vi "Convert String To Ring.vi"(8 "error in (no error)":errorcluster, 10 "Value":string, 11 "Ring Refnum":refnum<vi>) -> (0 "error out":errorcluster)   [LabVIEW 2013]
panel:
  in  "Numeric":u32
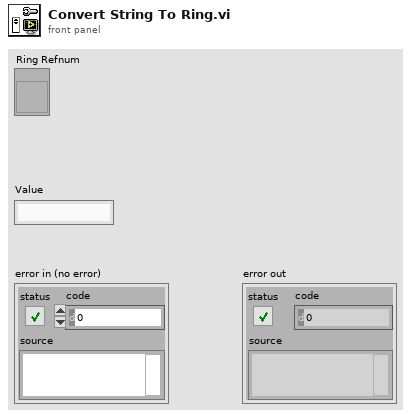
[diagram p1: front panel]
types:
  T1 = typedef "LVStringsAndValuesArrayTypeDef.ctl" = cluster{"String":string, "Value":ext}[]
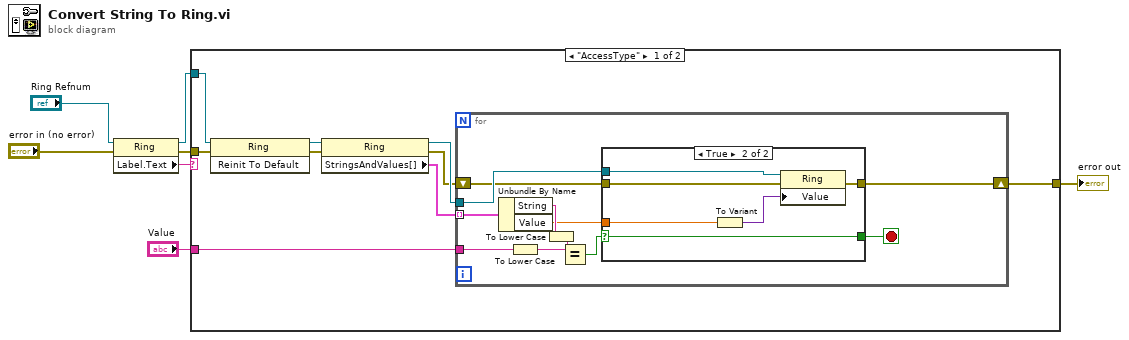
[diagram p0: block diagram]
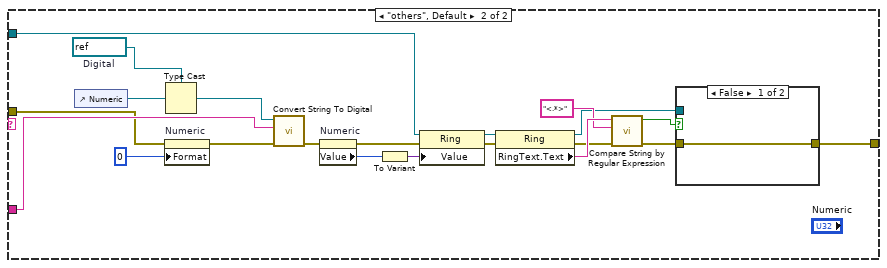
[diagram p3: hidden frame]
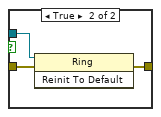
[diagram p4: hidden frame]
diagram:
  n1 = property class="Ring"(reference="Ring Refnum", error in="error in (no error)") -> (reference out=w4:refnum<vi>, error out=w2:errorcluster, "Label.Text"=w1:string)
  n2 = case shown="\"AccessType\"" w1 {
    tunnel: "Value" -> [w15 w56]
    tunnel: [w8 w43] -> w7
    tunnel: w2 -> [w13 w38]
    tunnel: w4 -> [w14 w36]
    frame "AccessType" {
      n3 = invoke class="Ring" method="Reinit To Default"(reference=w14, error in=w13) -> (reference out=w11:refnum<vi>, error out=w12:errorcluster)  [unwired: 1 in, 1 out]
      n4 = property class="Ring"(reference=w11, error in=w12) -> (reference out=w10:refnum<vi>, error out=w9:errorcluster, "StringsAndValues[]"=w16:T1)
      n5 = for {
        tunnel: w16 -> [w27] mode=indexing
        tunnel: w15 -> [w26]
        tunnel: w10 -> [w20]
        shift-right: [w18] -> w8
        shift-left: w9 -> [w19]
        stop <- w22 stop-if-true
        n6 = Unbundle By Name(w27) -> ("String"=w24:string, "Value"=w21:ext)
        n7 = To Lower Case(string=w26) -> (all lower case string=w25:string)
        n8 = To Lower Case(string=w24) -> (all lower case string=w17:string)
        n9 = Equal?(x=w25, y=w17) -> (x = y?=w23:bool)
        n10 = case shown="True" w23 {
          selector: w23 -> [w29 w35]
          tunnel: [w29 w35] -> w22
          tunnel: w21 -> [_ w31]
          tunnel: w20 -> [_ w34]
          tunnel: w19 -> [w28 w33]
          tunnel: [w28 w30] -> w18
          frame False {
          }
          frame True {
            n11 = To Variant(anything=w31) -> (Variant=w32:variant)
            n12 = property class="Ring"(reference=w34, error in=w33, "Value"=w32) -> (error out=w30:errorcluster)  [unwired: 1 out]
          }
        }
      }
    }
    frame "others", Default {
      w53 = refnum<vi> refnum  # Digital
      n13 = control-ref of="Numeric"() -> (w55:refnum<vi>)
      n14 = property on="Numeric" class="DigNum (strict)"(error in=w38, "Format"=u8 0 ("Display Format:Format")) -> (error out=w37:errorcluster)  [unwired: 1 in, 1 out]
      n15 = Type Cast(type=w53, x=w55) -> (*(type *) &x=w54:refnum<vi>)
      n16 = call "Convert String To Digital.vi"("error in (no error)"=w37, "Value"=w56, "DigNum Refnum"=w54) -> ("error out"=w52:errorcluster)  [unwired: 8 in]
      n17 = property on="Numeric" class="DigNum (strict)"(error in=w52) -> (error out=w40:errorcluster, "Value"=w42:u32)  [unwired: 1 in, 1 out]
      n18 = To Variant(anything=w42) -> (Variant=w41:variant)
      n19 = property class="Ring"(reference=w36, error in=w40, "Value"=w41) -> (reference out=w50:refnum<vi>, error out=w51:errorcluster)
      n20 = property class="Ring"(reference=w50, error in=w51) -> (reference out=w44:refnum<vi>, error out=w48:errorcluster, "RingText.Text"=w49:string)
      n21 = call "Compare String by Regular Expression.vi"("error in"=w48, "regular expression"="<.*>", "String"=w49) -> ("error out"=w45:errorcluster, "x = y?"=w46:bool)  [unwired: 7 in]
      n22 = case shown="False" w46 {
        tunnel: w45 -> [w57 w60]
        tunnel: w44 -> [_ w59]
        tunnel: [w57 w58] -> w43
        frame False {
        }
        frame True {
          n23 = invoke class="Ring" method="Reinit To Default"(reference=w59, error in=w60) -> (error out=w58:errorcluster)  [unwired: 1 in, 2 out]
        }
      }
    }
  }
  "error out" <- w7
